vi "stoper.vi"(9 "start":bool, 11 "x mission":dbl) -> (1 "frome start":u32, 2 "x rate":dbl, 3 "loop":u32)   [LabVIEW 2021]
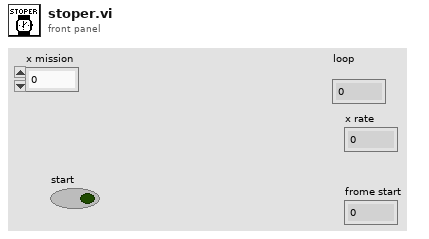
[diagram p1: front panel]
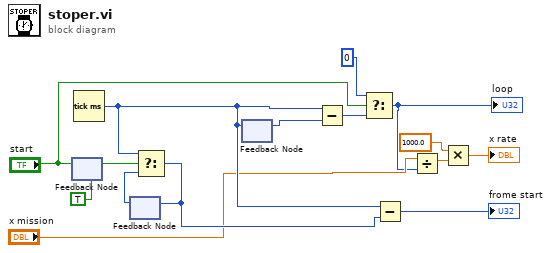
[diagram p0: block diagram]
diagram:
  n1 = feedback #1(TRUE) -> (w12:bool)
  n2 = feedback-in #1("start") -> ()
  n3 = Tick Count (ms)() -> (millisecond timer value=w14:u32)
  n4 = feedback #2() -> (w11:u32)  [unwired: 1 in]
  n5 = Select(t=w14, s=w12, f=w11) -> (s? t:f=w15:u32)
  n6 = feedback-in #2(w15) -> ()
  n7 = feedback #3() -> (w9:u32)  [unwired: 1 in]
  n8 = feedback-in #3(w14) -> ()
  n9 = Subtract(x=w14, y=w9) -> (x-y=w8:u32)
  n10 = Select(t=u32 0, s="start", f=w8) -> (s? t:f=w2:u32)
  "loop" <- w2
  n11 = Subtract(x=w14, y=w15) -> (x-y=→"frome start":u32)
  n12 = Divide(x="x mission", y=w2) -> (x/y=w5:dbl)
  n13 = Multiply(x=1000.0, y=w5) -> (x*y=→"x rate":dbl)
